vi "lab-project-vi.vi"() -> ()   [LabVIEW 2024]
panel:
  out "Time (s)":dbl
  out "T(C)":dbl
  out "T(K)":dbl
  in  "stop":bool
  out "Resistance":dbl
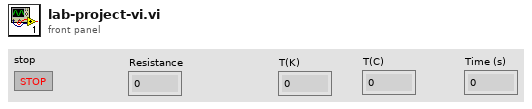
[diagram p1: front panel]
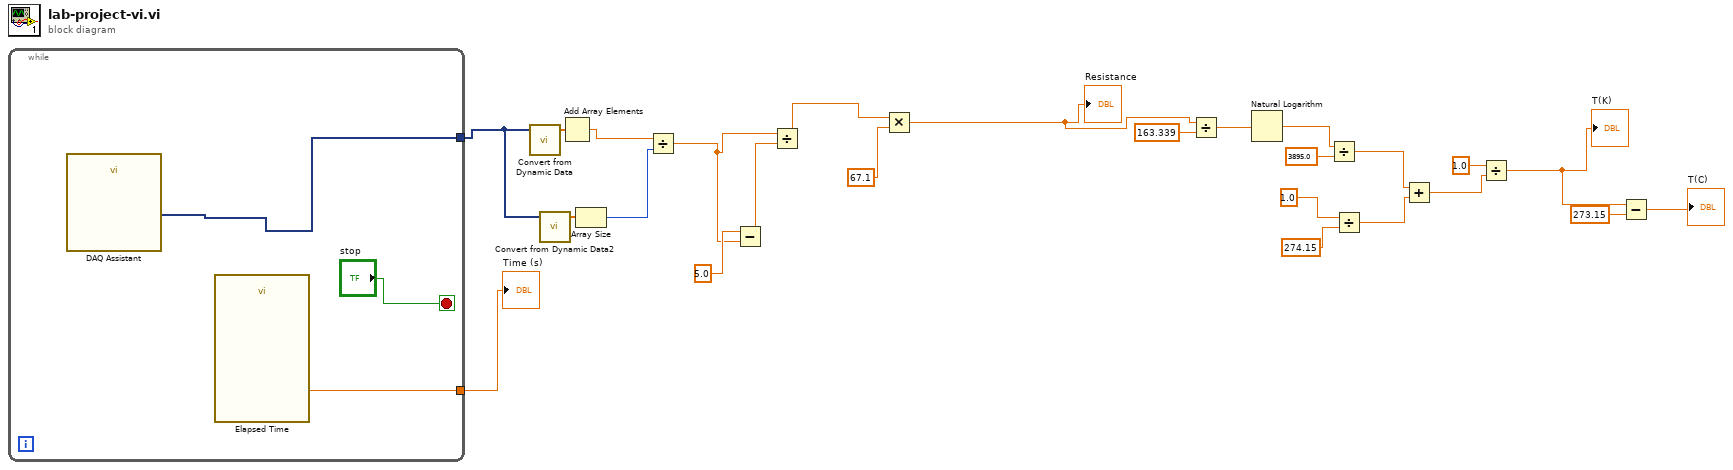
[diagram p0: block diagram]
diagram:
  n1 = while {
    tunnel: [w27] -> w24
    tunnel: [w26] -> w1
    stop <- "stop" stop-if-true
    n2 = call "DAQ Assistant"() -> ("data"=w27:dynamicdata)  [unwired: 17 in, 2 out]
    n3 = call "Elapsed Time"() -> ("Elapsed Time (s)"=w26:dbl)  [unwired: 12 in, 7 out]
  }
  "Time (s)" <- w1
  n4 = call "Convert from Dynamic Data"("Dynamic Data Type"=w24) -> ("Array"=w25:dbl[])  [unwired: 3 in]
  n5 = call "Convert from Dynamic Data2"("Dynamic Data Type"=w24) -> ("Array"=w23:dbl[])  [unwired: 3 in]
  n6 = Add Array Elements(numeric array=w25) -> (sum=w21:dbl)
  n7 = Array Size(array=w23) -> (size(s)=w22:i32)
  n8 = Divide(x=w21, y=w22) -> (x/y=w18:dbl)
  n9 = Subtract(x=5.0, y=w18) -> (x-y=w19:dbl)
  n10 = Divide(x=w18, y=w19) -> (x/y=w17:dbl)
  n11 = Multiply(x=w17, y=67.1) -> (x*y=w15:dbl)
  "Resistance" <- w15
  n12 = Divide(x=w15, y=163.339) -> (x/y=w13:dbl)
  n13 = Natural Logarithm(1:w13) -> (0:w12:dbl)
  n14 = Divide(x=w12, y=3895.0) -> (x/y=w7:dbl)
  n15 = Divide(x=1.0, y=274.15) -> (x/y=w8:dbl)
  n16 = Add(x=w7, y=w8) -> (x+y=w5:dbl)
  n17 = Divide(x=1.0, y=w5) -> (x/y=w4:dbl)
  "T(K)" <- w4
  n18 = Subtract(x=w4, y=273.15) -> (x-y=→"T(C)":dbl)
